vi "Get All Incoming Frames.vi"(8 "error in":errorcluster, 11 "Item Ref":T3 format="%.0x") -> (0 "error out":errorcluster, 2 "Frames":T2(array[cluster]), 3 "Item Ref out":T3 format="%.0x")   [LabVIEW 2023, in "J1939 Addon System Explorer.lvlib"]
uses:
  J1939 Addon System Explorer.lvlib
  <vilib>/NI VeriStand/Custom Device API/Custom Device Item Ref.ctl
  Addon Shared/Types/SPN Properties.ctl
  Addon Shared/SubVIs/Constants.vi
  <vilib>/NI VeriStand/Custom Device Tools/Custom Device Utility Library/NI VeriStand - Search for All Items by GUID.vi
  <vilib>/NI VeriStand/Custom Device API/Get Item Property (U32).vi
  <vilib>/NI VeriStand/Custom Device API/Get Item Property (Variant).vi
  Addon Shared/J1939 Addon Shared.lvlib
  <vilib>/NI VeriStand/Custom Device Tools/Custom Device Utility Library/Custom Device Utility Library.lvlib
  <vilib>/NI VeriStand/Custom Device API/Custom Device API.lvlib
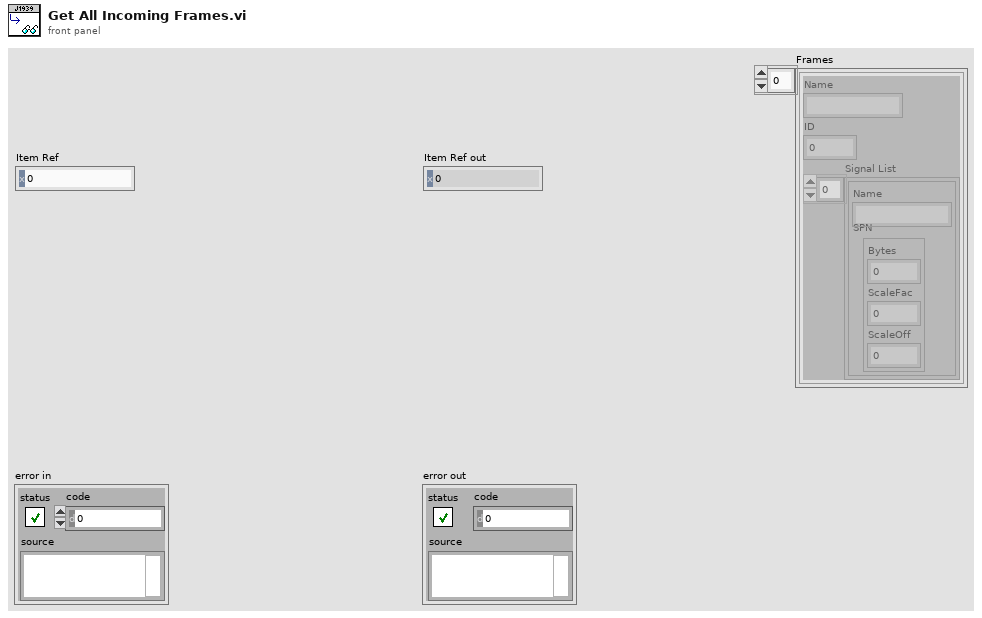
[diagram p1: front panel]
types:
  T1 = typedef "J1939 Addon Shared.lvlib/SPN Properties.ctl" = cluster{"Bytes":u32, "ScaleFac":dbl, "ScaleOff":dbl}
  T2 = cluster{"Name":string, "ID":u32, "Signal List":cluster{"Name":string, "SPN":T1}[]}[]
  T3 = typedef "Custom Device API.lvlib/Custom Device Item Ref.ctl" = u64
  T4 = typedef "Custom Device API.lvlib/Custom Device Item Info.ctl" = cluster{"Name":string, "Is Channel":bool, "GUID":string, "Is Waveform":bool}
  T5 = cluster{"Name":string, "Value":u32, cluster{"Name":string, "cluster":T1}[]}
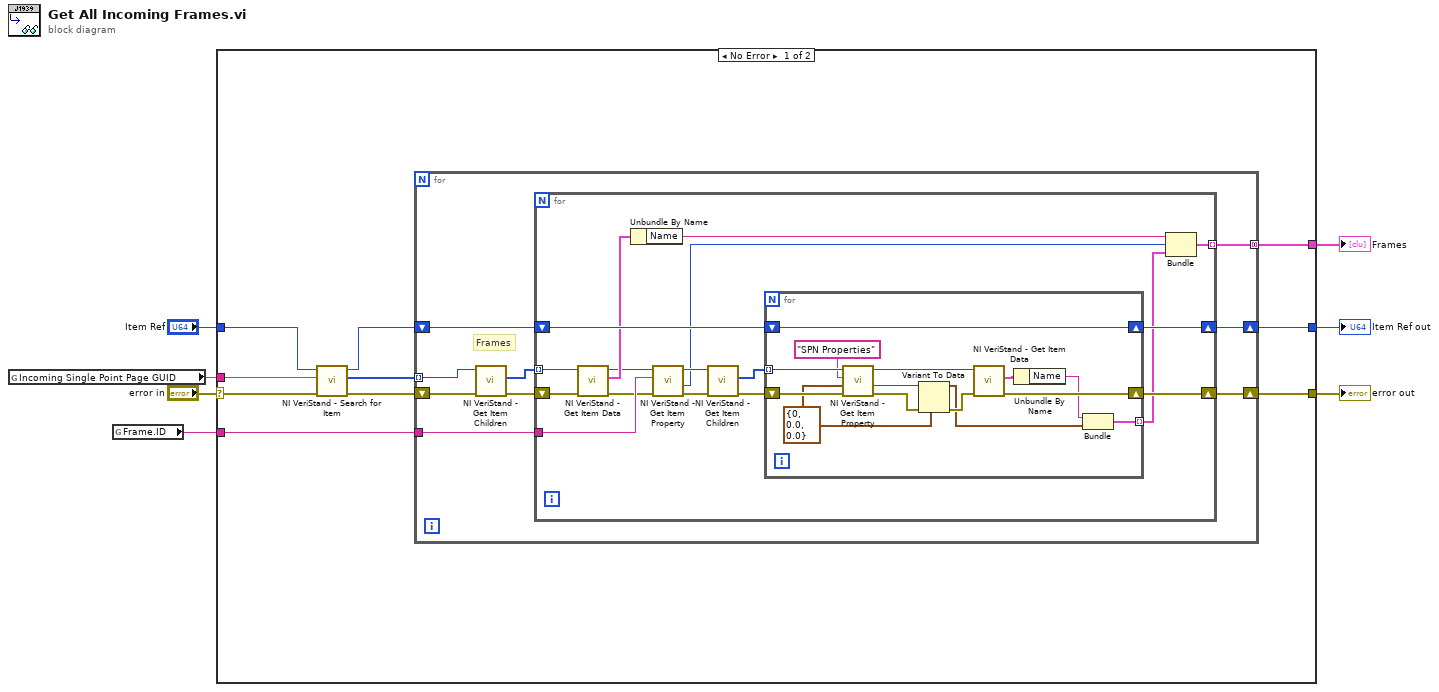
[diagram p0: block diagram]
diagram:
  n1 = global read "Constants.vi" "Incoming Single Point Page GUID"() -> (w3:string)
  n2 = global read "Constants.vi" "Frame.ID"() -> (w6:string)
  n3 = case shown="No Error" "error in" {
    selector: "error in" -> [w12 w59]
    tunnel: [w14 w58] -> w7
    tunnel: w6 -> [w17 _]
    tunnel: [w13 w59] -> w5
    tunnel: "Item Ref" -> [w10 w58]
    tunnel: w3 -> [w11 _]
    tunnel: [w8 _] -> w1
    frame No Error {
      n4 = call-poly <vilib>:"NI VeriStand - Search for Item.vi"("error in"=w12, "Item GUID"=w11, "Section Ref in"=w10) -> ("error out"=w16:errorcluster, "Item Refs"=w15:T3[], "Section Ref out"=w9:T3)  [unwired: 5 in, 1 out]
      n5 = for {
        tunnel: w17 -> [w26]
        tunnel: w15 -> [w23] mode=indexing
        tunnel: [w19] -> w8 mode=concatenating
        shift-right: [w22] -> w14
        shift-left: w9 -> [w18]
        shift-right: [w20] -> w13
        shift-left: w16 -> [w24]
        # "Frames"
        n6 = call <vilib>:"NI VeriStand - Get Item Children.vi"("error in (no error)"=w24, "Item Ref in"=w23) -> ("error out"=w21:errorcluster, "Child Refs"=w25:T3[])  [unwired: 6 in, 2 out]
        n7 = for {
          shift-right: [w30] -> w20
          shift-left: w21 -> [w35]
          tunnel: w25 -> [w36] mode=indexing
          tunnel: w26 -> [w43]
          shift-right: [w38] -> w22
          shift-left: w18 -> [w39]
          tunnel: [w31] -> w19 mode=indexing
          n8 = call <vilib>:"NI VeriStand - Get Item Data.vi"("error in (no error)"=w35, "Item Ref in"=w36) -> ("error out"=w32:errorcluster, "Item Info"=w34:T4, "Item Ref out"=w33:T3)  [unwired: 6 in, 1 out]
          n9 = Unbundle By Name(w34) -> ("Name"=w28:string)
          n10 = call-poly <vilib>:"NI VeriStand - Get Item Property.vi"("error in (no error)"=w32, "Property Name"=w43, "Item Ref in"=w33) -> ("error out"=w42:errorcluster, "Value"=w29:u32, "Item Ref out"=w41:T3)  [unwired: 5 in, 1 out]
          n11 = call <vilib>:"NI VeriStand - Get Item Children.vi"("error in (no error)"=w42, "Item Ref in"=w41) -> ("error out"=w40:errorcluster, "Child Refs"=w37:T3[])  [unwired: 6 in, 2 out]
          n12 = for {
            shift-right: [w54] -> w30
            shift-left: w40 -> [w50]
            tunnel: w37 -> [w57] mode=indexing
            shift-right: [w55] -> w38
            shift-left: w39 -> [w55]
            tunnel: [w47] -> w27 mode=indexing
            w46 = T1 {"Bytes"=0, "ScaleFac"=0.0, "ScaleOff"=0.0} ("cluster")
            n13 = call-poly <vilib>:"NI VeriStand - Get Item Property.vi"("error in (no error)"=w50, "Default Value"=w46, "Property Name"="SPN Properties" ("SPN Properties"), "Item Ref in"=w57) -> ("error out"=w49:errorcluster, "Value"=w51:variant, "Item Ref out"=w53:T3)  [unwired: 4 in, 1 out]
            n14 = Variant To Data(error in=w49, type=w46, Variant=w51) -> (data=w45:T1, error out=w52:errorcluster)
            n15 = call <vilib>:"NI VeriStand - Get Item Data.vi"("error in (no error)"=w52, "Item Ref in"=w53) -> ("error out"=w54:errorcluster, "Item Info"=w56:T4)  [unwired: 6 in, 2 out]
            n16 = Unbundle By Name(w56) -> ("Name"=w48:string)
            n17 = Bundle("Name"=w48, "cluster"=w45) -> (w47:cluster{"Name":string, "cluster":T1})  [unwired: 1 in]
          }
          n18 = Bundle("Name"=w28, "Value"=w29, w27) -> (w31:T5)  [unwired: 1 in]
        }
      }
    }
    frame Error {
    }
  }
  "error out" <- w5
  "Item Ref out" <- w7
  "Frames" <- w1
